vi "FLIN Init.vi"(9 "BaudRate":i32, 10 "LINIndex":u8, 11 "DevHandle":i32) -> (3 "function return":i32)   [LabVIEW 2010, in "usb2fast_lin.lvlib"]
doc: "int WINAPI FLIN_Init(int DevHandle,unsigned char LINIndex,int BaudRate);"
uses:
  usb2fast_lin.lvlib
  USB2XXX/trunk/USB2XXX/USB2XXX/vs2010/Release/USB2XXX.dll
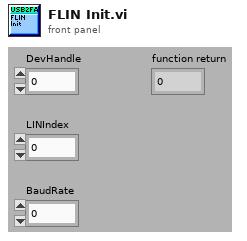
[diagram p1: front panel]
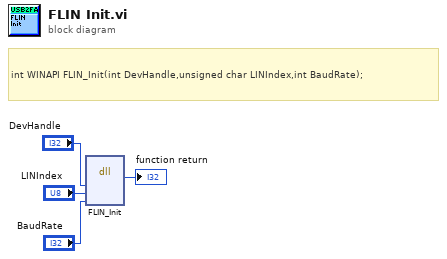
[diagram p0: block diagram]
diagram:
  # "int WINAPI FLIN_Init(int DevHandle,unsigned char LINIndex,int BaudRate);"
  n1 = dll-call lib="E:/Projects/USB2XXX/trunk/USB2XXX/USB2XXX/vs2010/Release/USB2XXX.*" fn="FLIN_Init"("DevHandle"="DevHandle", "LINIndex"="LINIndex", "BaudRate"="BaudRate") -> (→"function return":i32)  [unwired: 6 in, 2 out]
